vi "Error Write Status.vi"(8 "error in":errorcluster, 10 "Error STS":i32[](array[numeric]), 11 "Error in":refnum<class "Error.lvclass">) -> (0 "error out":errorcluster, 3 "Error out":refnum<class "Error.lvclass">)   [LabVIEW 2023, in "Error.lvclass"]
uses:
  Error.lvclass
  Error.lvclass/Error.ctl
  <vilib>/ADAS Replay HIL/Channels/Tag Wrapper/Polymorphic/Write Channel (I32).vi/cccb8e89-591f-4bb4-9d4e-ae06ba1f5498.vi
  <vilib>/ADAS Replay HIL/Channels/Tag Wrapper/Polymorphic/Write Channel (I32).vi/cccb8e89-591f-4bb4-9d4e-ae06ba1f5498.vi/4bc1c15b-36ab-481f-b8dd-c64075ce723a.vi
  <vilib>/ADAS Replay HIL/Channels/Tag Wrapper/Polymorphic/Write Channel (I32).vi/cccb8e89-591f-4bb4-9d4e-ae06ba1f5498.vi/d83cb72b-7713-41fc-a3d1-682de79cf574.vi
  <vilib>/ADAS Replay HIL/Channels/Tag Wrapper/Polymorphic/Write Channel (I32).vi
  <vilib>/ADAS Replay HIL/Channels/Tag Wrapper/Tag Wrapper.lvlib
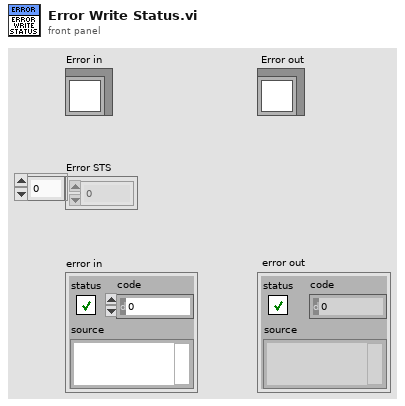
[diagram p1: front panel]
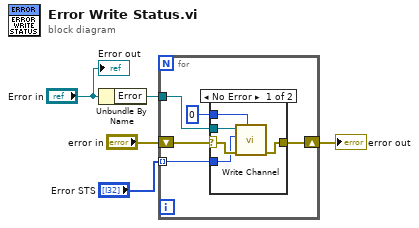
[diagram p0: block diagram]
diagram:
  n1 = Unbundle By Name("Error in") -> ("Error"=w5:refnum<k21>)
  n2 = for {
    tunnel: w5 -> [w10]
    tunnel: "Error STS" -> [w9] mode=indexing
    shift-right: [w7] -> w3
    shift-left: "error in" -> [w8]
    n3 = case shown="No Error" w8 {
      selector: w8 -> [w15 w16]
      tunnel: [w14 w16] -> w7
      tunnel: w10 -> [w13 _]
      tunnel: w9 -> [w12 _]
      tunnel: 0 ("Timeout (ms)") -> [w11 _]
      frame No Error {
        n4 = call-poly <vilib>:"Write Channel.vi"("Timeout (ms)"=w11, "error in"=w15, "Value to Write"=w12, "ADAS HIL Channel in"=w13) -> ("error out"=w14:errorcluster)  [unwired: 5 in, 2 out]
      }
      frame Error {
      }
    }
  }
  "error out" <- w3
  "Error out" <- "Error in"
